vi "Resource - IsEXE.vi"() -> (2 "Is EXE?":bool)   [LabVIEW 2020]
doc: "Is EXE?\nReturns TRUE if the environment is a runtime executable"
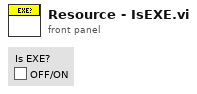
[diagram p1: front panel]
types:
  T1 = enum32{"invalid app kind", "Development System", "Run Time System", "Student Edition", "Embedded LabVIEW", "Evaluation", "Custom"}
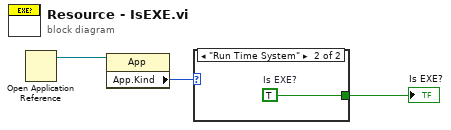
[diagram p0: block diagram]
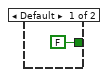
[diagram p2: hidden frame]
diagram:
  n1 = Open Application Reference() -> (3:w1:refnum<vi>)  [unwired: 4 in, 1 out]
  n2 = property class="App"(reference=w1) -> ("App.Kind"=w2:T1)  [unwired: 1 in, 2 out]
  n3 = case shown="\"Run Time System\"" w2 {
    tunnel: [FALSE ("Is EXE?") w5] -> w3
    frame Default {
    }
    frame "Run Time System" {
      w5 = TRUE  # Is EXE?
    }
  }
  "Is EXE?" <- w3
